vi "X in Y (Variant)__jki_lib_array -- VI Tester.vi"(1 "array":variant[](array[variant]), 2 "element":variant) -> (6 "element in array?":bool)   [LabVIEW 2011]
panel:
  # "Copyright © 2008 JKI. All rights reserved.\n\nAuthor: Jim Kring [jim.kring@jameskring.com]\n\nThis library is provided \"AS IS\" ,WITHOUT WARRANTIES OR \nCONDITIONS OF ANY KIND, either express or implied.\n\nJKI -- http://www.jameskring.com"
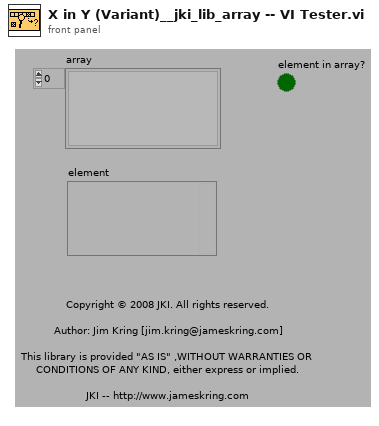
[diagram p1: front panel]
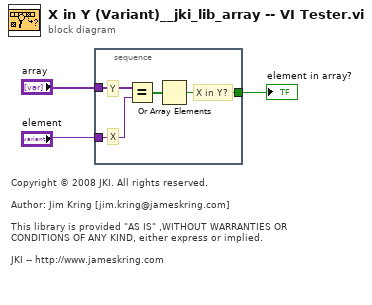
[diagram p0: block diagram]
diagram:
  # "Copyright © 2008 JKI. All rights reserved.\n\nAuthor: Jim Kring [jim.kring@jameskring.com]\n\nThis library is provided \"AS IS\" ,WITHOUT WARRANTIES OR \nCONDITIONS OF ANY KIND, either express or implied.\n\nJKI -- http://www.jameskring.com"
  n1 = stacked-sequence {
    tunnel: "element" -> [w7]
    tunnel: "array" -> [w6]
    tunnel: [w4] -> w3
    frame #0 {
      # "X in Y?"
      # "X"
      # "Y"
      n2 = Equal?(x=w6, y=w7) -> (x = y?=w5:bool[])
      n3 = Or Array Elements(Boolean array=w5) -> (logical OR=w4:bool)
    }
  }
  "element in array?" <- w3
